vi "Extractor Blobs.vi"() -> ()   [LabVIEW 2012]
doc: "Use this template to build a producer/consumer design pattern. Use this template when you need to execute a process, such as data analysis, when a data source, such as a triggered acquisition, produces data at an uneven rate and you need to execute the process when the data becomes available."
uses:
  <vilib>/vision/Image Controls.llb/IMAQ Image.ctl
  Global Variables.vi
  <vilib>/Utility/file.llb/Write To Spreadsheet File (string).vi
  <vilib>/vision/NI_Vision_Development_Module.lvlib
panel:
  out "blobNbr":i32
  out "outPath":path
  in  "Zoom out":bool
  out "TargVec1":string[](array[string])
  out "Targets":path
  out "Datos":path
  in  "Box size":i32(knob)=25 min=3 max=51 step=2 scale=3.0..51.0 scale format="%#.6g"
  in  "Aguacate":bool
  in  "Guardar":bool
  out "Image 2":T1(plugin-control)
  out "Cuadro":i32[](array[numeric])
  out "Image":T1(plugin-control)
  in  "Image\n  Path":path
  in  "stop":bool
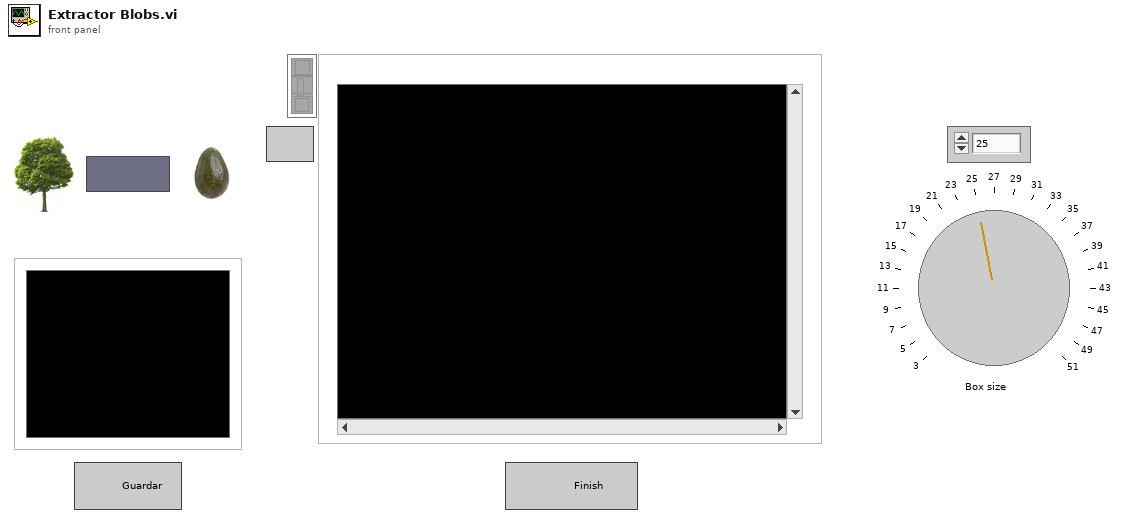
[diagram p1: front panel]
types:
  T1 = typedef "IMAQ Image.ctl" = refnum<image>
  T2 = typedef "Image Type" = u32
  T3 = enum16{"open", "replace", "create", "open or create", "replace or create", "replace or create with confirmation"}
  T4 = cluster{"Global Rectangle":i32[], "Contours":cluster{"Contour Type":u32, "ROI Type":u32, "Points":i32[]}[]}
  T5 = cluster{"Contour Type":u32, "ROI Type":u32, "Points":i32[]}[]
  T6 = cluster{"Contour Type":u32, "ROI Type":u32, "Points":i32[]}
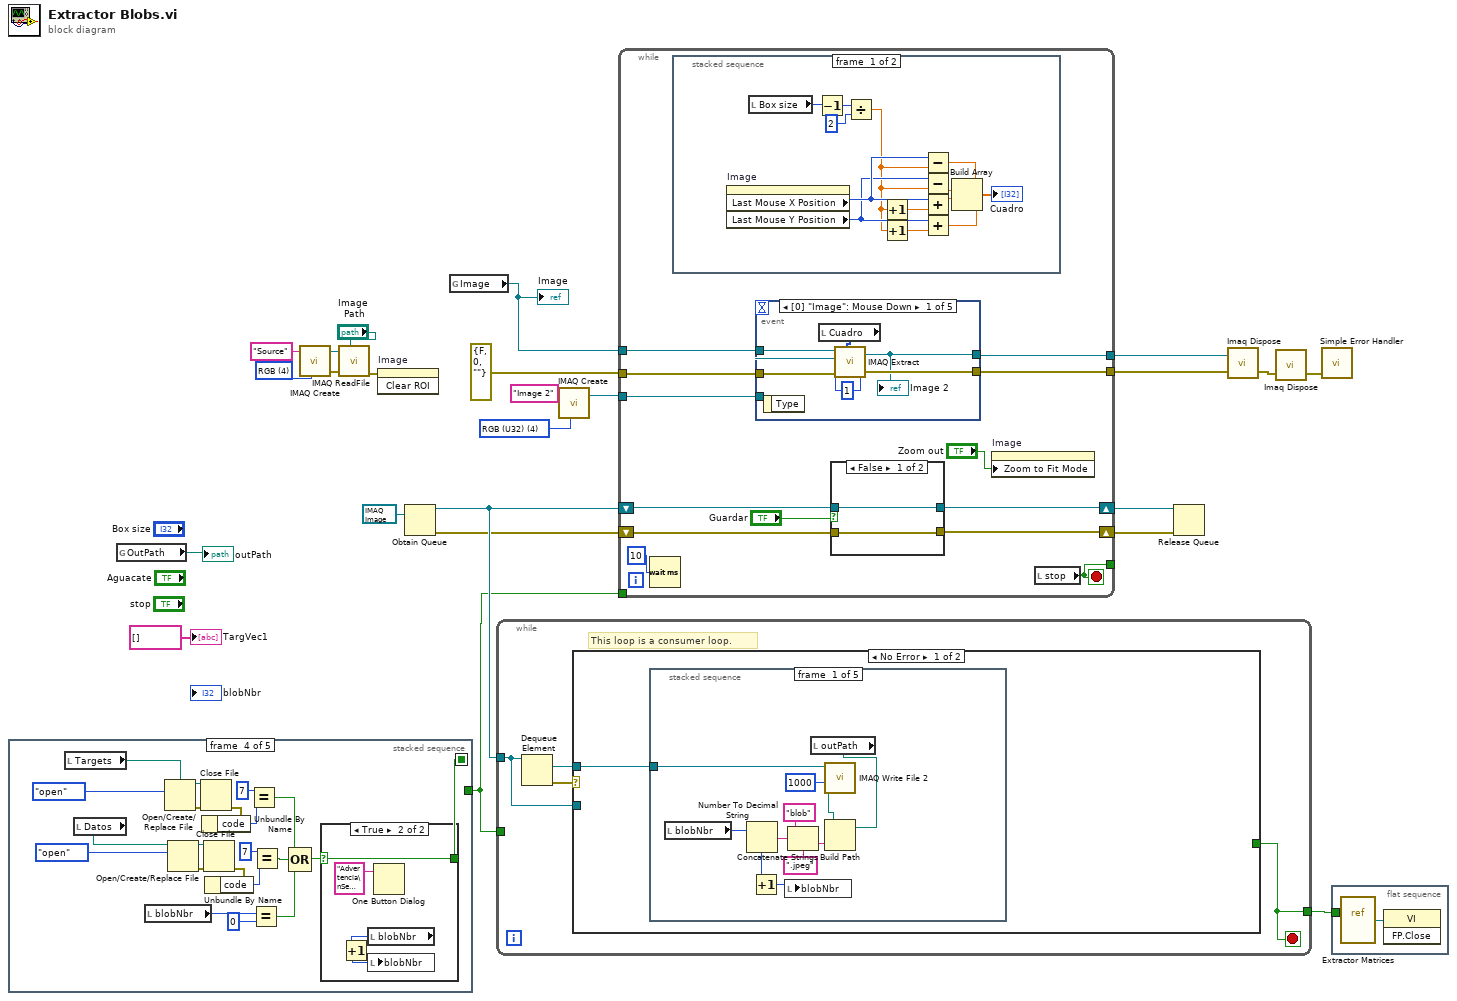
[diagram p0: block diagram]
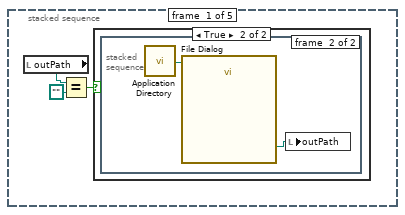
[diagram p2: hidden frame]
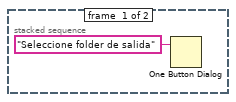
[diagram p4: hidden frame]
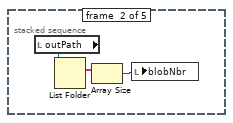
[diagram p5: hidden frame]
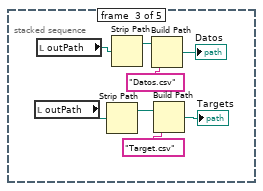
[diagram p6: hidden frame]
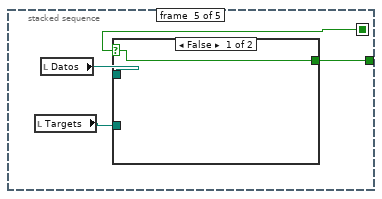
[diagram p8: hidden frame]
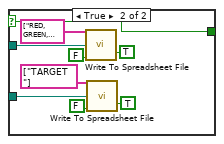
[diagram p9: hidden frame]
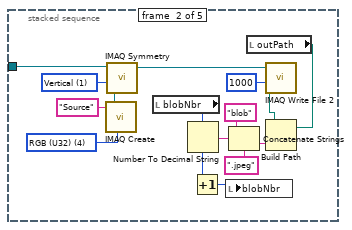
[diagram p10: hidden frame]
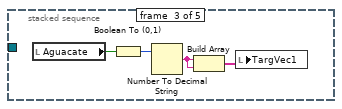
[diagram p11: hidden frame]
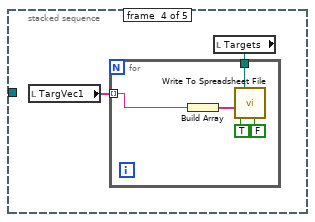
[diagram p12: hidden frame]
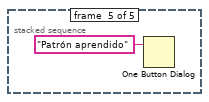
[diagram p13: hidden frame]
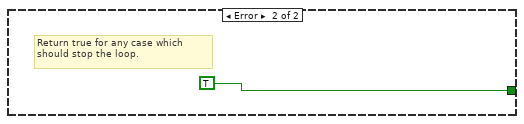
[diagram p14: hidden frame]
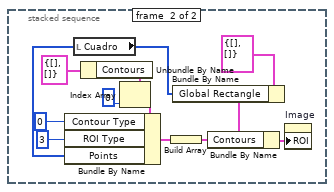
[diagram p15: hidden frame]
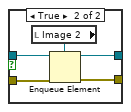
[diagram p16: hidden frame]
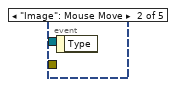
[diagram p17: hidden frame]
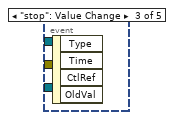
[diagram p18: hidden frame]
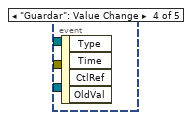
[diagram p19: hidden frame]
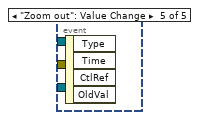
[diagram p20: hidden frame]
diagram:
  w4 = T2 4 items=["Grayscale (U8)", "Grayscale (I16)", "Grayscale (SGL)", "Complex (CSG)", "RGB (U32)", "HSL (U32)", "RGB (U64)", "Grayscale (U16)"] ("Image Type")
  w20 = u32 4 items=["8 bits", "16 bits", "Float", "Complex", "RGB", "HSL"] ("Image Type")
  n1 = stacked-sequence {
    seq-local: [_ _ _ w48 _] -> [_ _ _ _ w70]
    tunnel: [_ _ _ _ w68] -> w7
    frame #0 {
      n2 = local read "outPath"() -> (w25:path)
      n3 = Equal?(x=w25, y=path "") -> (x = y?=w27:bool)
      n4 = case shown="True" w27 {
        frame False {
        }
        frame True {
          n5 = stacked-sequence {
            frame #0 {
              n6 = One Button Dialog(message="Seleccione folder de salida") -> ()  [unwired: 1 in, 1 out]
            }
            frame #1 {
              n7 = call <vilib>:"Application Directory.vi"() -> ("Application Directory"=w29:path)
              n8 = call "File Dialog"("start path"=w29) -> ("selected path"=w30:path)  [unwired: 11 in, 3 out]
              n9 = local write "outPath"(w30) -> ()
            }
          }
        }
      }
    }
    frame #1 {
      n10 = local read "outPath"() -> (w33:path)
      n11 = List Folder(path=w33) -> (filenames=w32:string[])  [unwired: 3 in, 3 out]
      n12 = Array Size(array=w32) -> (size(s)=w31:i32)
      n13 = local write "blobNbr"(w31) -> ()
    }
    frame #2 {
      n14 = local read "outPath"() -> (w36:path)
      n15 = local read "outPath"() -> (w34:path)
      n16 = Strip Path(path=w36) -> (stripped path=w37:path)  [unwired: 1 out]
      n17 = Strip Path(path=w34) -> (stripped path=w35:path)  [unwired: 1 out]
      n18 = Build Path(base path=w35, name or relative path="Datos.csv") -> (appended path=→"Datos":path)
      n19 = Build Path(base path=w37, name or relative path="Target.csv") -> (appended path=→"Targets":path)
    }
    frame #3 {
      n20 = local read "Targets"() -> (w58:path)
      n21 = local read "Datos"() -> (w49:path)
      n22 = local read "blobNbr"() -> (w47:i32)
      n23 = Open/Create/Replace File(file path (use dialog)=w58, operation (0:open)=T3."open") -> (refnum out=w60:refnum<file>, error out=w61:errorcluster)  [unwired: 4 in, 1 out]
      n24 = Open/Create/Replace File(file path (use dialog)=w49, operation (0:open)=T3."open") -> (refnum out=w52:refnum<file>, error out=w51:errorcluster)  [unwired: 4 in, 1 out]
      n25 = Close File(refnum=w60, error in=w61) -> (error out=w59:errorcluster)  [unwired: 1 out]
      n26 = Unbundle By Name(w59) -> ("code"=w57:i32)
      n27 = Close File(refnum=w52, error in=w51) -> (error out=w53:errorcluster)  [unwired: 1 out]
      n28 = Unbundle By Name(w53) -> ("code"=w54:i32)
      n29 = Equal?(x=7 ("y"), y=w57) -> (x = y?=w45:bool)
      n30 = Equal?(x=w47, y=0) -> (x = y?=w42:bool)
      n31 = Equal?(x=7 ("y"), y=w54) -> (x = y?=w43:bool)
      n32 = Compound Arithmetic op=OR(w45, w43, w42) -> (w44:bool)
      n33 = case shown="True" w44 {
        selector: w44 -> [w63 w66]
        tunnel: [w63 w66] -> w48
        frame False {
        }
        frame True {
          n34 = local read "blobNbr"() -> (w65:i32)
          n35 = Increment(x=w65) -> (x+1=w64:i32)
          n36 = local write "blobNbr"(w64) -> ()
          n37 = One Button Dialog(message="Advertencia\nSe procederá a crear un archivo de\n patrones ") -> ()  [unwired: 1 in, 1 out]
        }
      }
    }
    frame #4 {
      n38 = local read "Targets"() -> (w69:path)
      n39 = local read "Datos"() -> (w71:path)
      n40 = case shown="False" w70 {
        selector: w70 -> [w72 w73]
        tunnel: w71 -> [_ w79]
        tunnel: w69 -> [_ w74]
        tunnel: [w72 w73] -> w68
        frame False {
        }
        frame True {
          n41 = call-poly <vilib>:"Write To Spreadsheet File.vi"("transpose? (no:F)"=TRUE, "append to file? (new file:F)"=FALSE, "1D data"=string[] ["RED,  GREEN, BLUE,    SAT, VAL "] ("appended array"), "file path (dialog if empty)"=w79) -> ()  [unwired: 4 in, 1 out]
          n42 = call-poly <vilib>:"Write To Spreadsheet File.vi"("transpose? (no:F)"=TRUE, "append to file? (new file:F)"=FALSE, "1D data"=string[] ["TARGET "] ("appended array"), "file path (dialog if empty)"=w74) -> ()  [unwired: 4 in, 1 out]
        }
      }
    }
  }
  n43 = global read "Global Variables.vi" "OutPath"() -> (→"outPath":path)
  n44 = call "IMAQ Create"("Image Name"="Source", "Image Type"=w20) -> ("New Image"=w17:T1, "error out"=w16:errorcluster)  [unwired: 2 in, 1 out]
  n45 = call "IMAQ ReadFile"("File Path"="Image\n  Path", "error in (no error)"=w16, "Image"=w17) -> ("error out"=w14:errorcluster)  [unwired: 2 in, 6 out]
  n46 = invoke on="Image" class="ImageControl" method="Clear ROI"(error in=w14) -> ()  [unwired: 2 in, 3 out]
  n47 = Obtain Queue(element data type=T1 refnum ("Image")) -> (queue out=w24:refnum<queue>, error out=w23:errorcluster)  [unwired: 4 in, 1 out]
  n48 = global read "Global Variables.vi" "Image"() -> (w5:T1)
  "Image" <- w5
  n49 = while {
    tunnel: w24 -> [w83]
    tunnel: w7 -> [_]
    tunnel: [w82] -> w6
    stop <- w82 stop-if-true
    # "This loop is a consumer loop."
    n50 = Dequeue Element(queue=w83) -> (element=w84:T1, error out=w85:errorcluster)  [unwired: 2 in, 2 out]
    n51 = case shown="No Error" w85 {
      tunnel: w84 -> [w86 _]
      tunnel: [_ TRUE] -> w82
      tunnel: w83 -> [_ _]
      frame No Error {
        n52 = stacked-sequence {
          tunnel: w86 -> [w95 w100 _ _ _]
          frame #0 {
            n53 = local read "blobNbr"() -> (w88:i32)
            n54 = Number To Decimal String(number=w88) -> (decimal integer string=w90:string)  [unwired: 1 in]
            n55 = Increment(x=w88) -> (x+1=w89:i32)
            n56 = local write "blobNbr"(w89) -> ()
            n57 = Concatenate Strings("blob" ("string"), w90, ".jpeg") -> (w91:string)
            n58 = local read "outPath"() -> (w87:path)
            n59 = Build Path(base path=w87, name or relative path=w91) -> (appended path=w94:path)
            n60 = call-poly "IMAQ Write File 2"("Image Quality"=u32 1000, "File Path"=w94, "Image"=w95) -> ()  [unwired: 7 in, 2 out]
          }
          frame #1 {
            w97 = u32 1 items=["Horizontal", "Vertical", "Central", "1st Diagonal", "2nd Diagonal"] ("Type of Symmetry")
            w99 = T2 4 items=["Grayscale (U8)", "Grayscale (I16)", "Grayscale (SGL)", "Complex (CSG)", "RGB (U32)", "HSL (U32)", "RGB (U64)", "Grayscale (U16)"] ("Image Type")
            n61 = call "IMAQ Create"("Image Name"="Source", "Image Type"=w99) -> ("New Image"=w101:T1)  [unwired: 2 in, 2 out]
            n62 = call "IMAQ Symmetry"("Type of Symmetry"=w97, "Image Dst"=w101, "Image Src"=w100) -> ("Image Dst Out"=w103:T1)  [unwired: 2 in, 1 out]
            n63 = local read "blobNbr"() -> (w104:i32)
            n64 = Number To Decimal String(number=w104) -> (decimal integer string=w106:string)  [unwired: 1 in]
            n65 = Increment(x=w104) -> (x+1=w105:i32)
            n66 = local write "blobNbr"(w105) -> ()
            n67 = Concatenate Strings("blob" ("string"), w106, ".jpeg") -> (w107:string)
            n68 = local read "outPath"() -> (w98:path)
            n69 = Build Path(base path=w98, name or relative path=w107) -> (appended path=w110:path)
            n70 = call-poly "IMAQ Write File 2"("Image Quality"=u32 1000, "File Path"=w110, "Image"=w103) -> ()  [unwired: 7 in, 2 out]
          }
          frame #2 {
            n71 = local read "Aguacate"() -> (w115:bool)
            n72 = Boolean To (0,1)(Boolean=w115) -> (0, 1=w114:i16)
            n73 = Number To Decimal String(number=w114) -> (decimal integer string=w112:string)  [unwired: 1 in]
            n74 = Build Array(w112, w112) -> (w113:string[])
            n75 = local write "TargVec1"(w113) -> ()
          }
          frame #3 {
            n76 = local read "TargVec1"() -> (w116:string[])
            n77 = local read "Targets"() -> (w117:path)
            n78 = for {
              tunnel: w116 -> [w118] mode=indexing
              tunnel: w117 -> [w119]
              n79 = Build Array(w118) -> (w120:string[])
              n80 = call-poly <vilib>:"Write To Spreadsheet File.vi"("transpose? (no:F)"=FALSE, "append to file? (new file:F)"=TRUE, "1D data"=w120, "file path (dialog if empty)"=w119) -> ()  [unwired: 4 in, 1 out]
            }
          }
          frame #4 {
            n81 = One Button Dialog(message="Patrón aprendido") -> ()  [unwired: 1 in, 1 out]
          }
        }
      }
      frame Error {
        # "Return true for any case which should stop the loop."
      }
    }
  }
  n82 = call "IMAQ Create"("Image Name"="Image 2", "Image Type"=w4) -> ("New Image"=w10:T1)  [unwired: 2 in, 2 out]
  n83 = while {
    shift-right: [w130] -> w21
    shift-left: w23 -> [w128]
    shift-right: [w131] -> w22
    shift-left: w24 -> [w129]
    tunnel: errorcluster {"status"=FALSE, "code"=0, "source"=""} ("error out") -> [w134]
    tunnel: w10 -> [w135]
    tunnel: w5 -> [w136]
    tunnel: [w133] -> w9
    tunnel: [w132] -> w8
    tunnel: w7 -> [_]
    tunnel: [w127] -> _
    stop <- w127 stop-if-true
    n84 = Wait (ms)(milliseconds to wait=u32 10) -> ()  [unwired: 1 out]
    n85 = stacked-sequence {
      frame #0 {
        n86 = property on="Image" class="ImageControl"() -> ("Last Mouse X Position"=w150:i32, "Last Mouse Y Position"=w149:i32)  [unwired: 2 in, 2 out]
        n87 = local read "Box size"() -> (w143:i32)
        n88 = Decrement(x=w143) -> (x-1=w142:i32)
        n89 = Divide(x=w142, y=2) -> (x/y=w138:dbl)
        n90 = Increment(x=w138) -> (x+1=w140:dbl)
        n91 = Increment(x=w138) -> (x+1=w139:dbl)
        n92 = Subtract(x=w150, y=w138) -> (x-y=w147:dbl)
        n93 = Subtract(x=w149, y=w138) -> (x-y=w148:dbl)
        n94 = Add(x=w150, y=w140) -> (x+y=w145:dbl)
        n95 = Add(x=w149, y=w139) -> (x+y=w144:dbl)
        n96 = Build Array(w147, w148, w145, w144) -> (→"Cuadro":dbl[])
      }
      frame #1 {
        n97 = local read "Cuadro"() -> (w158:i32[])
        n98 = Unbundle By Name(T4 {"Global Rectangle"=[], "Contours"=[]} ("ROI")) -> ("Contours"=w162:T5)
        n99 = Index Array(array=w162, index=0) -> (element=w160:T6)
        n100 = Bundle By Name(cluster=w160, "Contour Type"=0 ("index"), "ROI Type"=u32 3, "Points"=w158) -> (w156:T6)
        n101 = Build Array(w156) -> (w155:T5)
        n102 = Bundle By Name(cluster=T4 {"Global Rectangle"=[], "Contours"=[]} ("ROI"), "Global Rectangle"=w158) -> (w157:T4)
        n103 = Bundle By Name(cluster=w157, "Contours"=w155) -> (w152:T4)
        n104 = property on="Image" class="ImageControl"("ROI"=w152) -> ()  [unwired: 2 in, 2 out]
      }
    }
    n105 = event shown="[0] \"Image\": Mouse Down" {
      selector: _ -> [_ _ _ _ _]
      dyn-events: _ -> [_ _ _ _ _]
      timeout: _ -> [_ _ _ _ _]
      tunnel: w136 -> [w174 _ _ _ _]
      tunnel: w135 -> [w173 _ _ _ _]
      tunnel: w134 -> [w172 _ _ _ _]
      tunnel: [w170 _ _ _ _] -> w133
      tunnel: [w171 _ _ _ _] -> w132
      event "Image": Mouse Down {
        w175 = u32 1 ("Y Step")
        n106 = event-data() -> ()  [unwired: 1 in, 1 out]
        n107 = local read "Cuadro"() -> (w176:i32[])
        n108 = call "IMAQ Extract"("Y Step Size"=w175, "Optional Rectangle"=w176, "error in (no error)"=w172, "X Step Size"=w175, "Image Dst"=w173, "Image Src"=w174) -> ("error out"=w171:errorcluster, "Image Dst Out"=w170:T1)  [unwired: 4 out]
        "Image 2" <- w170
      }
      event "Image": Mouse Move {
        n109 = event-data() -> ()  [unwired: 1 in, 1 out]
      }
      event "stop": Value Change {
        n110 = event-data() -> ()  [unwired: 1 in, 4 out]
      }
      event "Guardar": Value Change {
        n111 = event-data() -> ()  [unwired: 1 in, 4 out]
      }
      event "Zoom out": Value Change {
        n112 = event-data() -> ()  [unwired: 1 in, 4 out]
      }
    }
    n113 = case shown="False" "Guardar" {
      tunnel: [w164 w169] -> w131
      tunnel: [w163 w168] -> w130
      tunnel: w129 -> [w164 w167]
      tunnel: w128 -> [w163 w166]
      frame False {
      }
      frame True {
        n114 = local read "Image 2"() -> (w165:T1)
        n115 = Enqueue Element(queue=w167, element=w165, error in (no error)=w166) -> (queue out=w169:refnum<queue>, error out=w168:errorcluster)  [unwired: 1 in, 1 out]
      }
    }
    n116 = property on="Image" class="ImageControl"("Zoom to Fit Mode"="Zoom out") -> ()  [unwired: 2 in, 2 out]
    n117 = local read "stop"() -> (w127:bool)
  }
  n118 = Release Queue(queue=w22, error in (no error)=w21) -> ()  [unwired: 1 in, 3 out]
  n119 = call "Imaq Dispose"("Image"=w9, "error in (no error)"=w8) -> ("error out"=w12:errorcluster)  [unwired: 1 in, 3 out]
  n120 = call "Imaq Dispose"("error in (no error)"=w12) -> ("error out"=w11:errorcluster)  [unwired: 2 in, 3 out]
  n121 = call <vilib>:"Simple Error Handler.vi"("error in (no error)"=w11) -> ()  [unwired: 1 in, 8 out]
  n122 = flat-sequence {
    tunnel: w6 -> [_]
    frame #0 {
      n123 = vi-ref "Extractor Matrices.vi"() -> (w177:refnum<vi>)
      n124 = invoke class="VI" method="FP.Close"(reference=w177) -> ()  [unwired: 2 in, 3 out]
    }
  }
  "TargVec1" <- string[] [] ("TargVec1")
